vi "Data Channel.vi"(8 "error in (no error)":errorcluster, 11 "Node Ptr":T2 format="%.0x") -> (0 "error out":errorcluster)   [LabVIEW 2019, in "RefMem DMA System Explorer.lvlib"]
uses:
  RefMem DMA System Explorer.lvlib
  <vilib>/NI VeriStand/Custom Device API/Custom Device Item Ref.ctl
  controls/Data Channel Type.ctl
  <vilib>/NI VeriStand/Custom Device API/Custom Device Channel Type.ctl
  Shared/Constants.vi
  <vilib>/NI VeriStand/Custom Device API/Get Item Property (U32).vi
  <vilib>/NI VeriStand/Custom Device API/Get Item Property (U16).vi
  <vilib>/NI VeriStand/Custom Device API/Set Item Property (U32).vi
  <vilib>/NI VeriStand/Custom Device API/Set Item Property (U16).vi
  <vilib>/NI VeriStand/Custom Device API/Custom Device API.lvlib
  Shared/RefMem DMA Shared.lvlib
panel:
  in  "Block Address":u32 format="%.0x"
  in  "Default Value":dbl
  in  "Unit":string
  in  "Warning text":string="WARNING: The address selected by this channel is within the range of addresses reserved by NI VeriStand's built in reflective memory support!"
  out "Warn Icon":bool
  in  "Type":T1
  in  "Relative offset in block":u32
  in  "Header":cluster{"Section Name":string}={"Section Name"="Data Channel"}
  in  "Description":string
  in  "Name":string
  # "In channels (doubles)"
  # "Channels to write has to be in row\nChannels to read can have space in between"
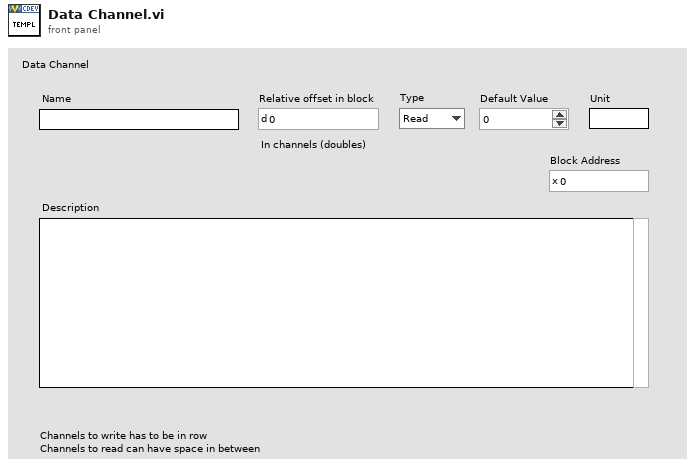
[diagram p1: front panel]
types:
  T1 = typedef "RefMem DMA System Explorer.lvlib/Data Channel Type.ctl" = enum16{"Read", "Write"}
  T2 = typedef "Custom Device API.lvlib/Custom Device Item Ref.ctl" = u64
  T3 = enum8{"Enabled", "Disabled", "Disabled and Grayed Out"}
  T4 = typedef "Custom Device API.lvlib/Custom Device Pointer.ctl" = refnum<k24>
  T5 = typedef "Custom Device API.lvlib/Custom Device Channel.ctl" = cluster{"Type":T6, "Units":string, "Default Value":dbl, "Faultable":bool, "Scalable":bool}
  T6 = typedef "Custom Device API.lvlib/Custom Device Channel Type.ctl" = enum16{"Input", "Output"}
  T7 = typedef "Custom Device API.lvlib/Custom Device Commands.ctl" = enum16{"Default", "Item renamed", "Shutdown", "Dynamic button pressed"}
  T8 = typedef "Custom Device API.lvlib/Custom Device Item Info.ctl" = cluster{"Name":string, "Is Channel":bool, "GUID":string, "Is Waveform":bool}
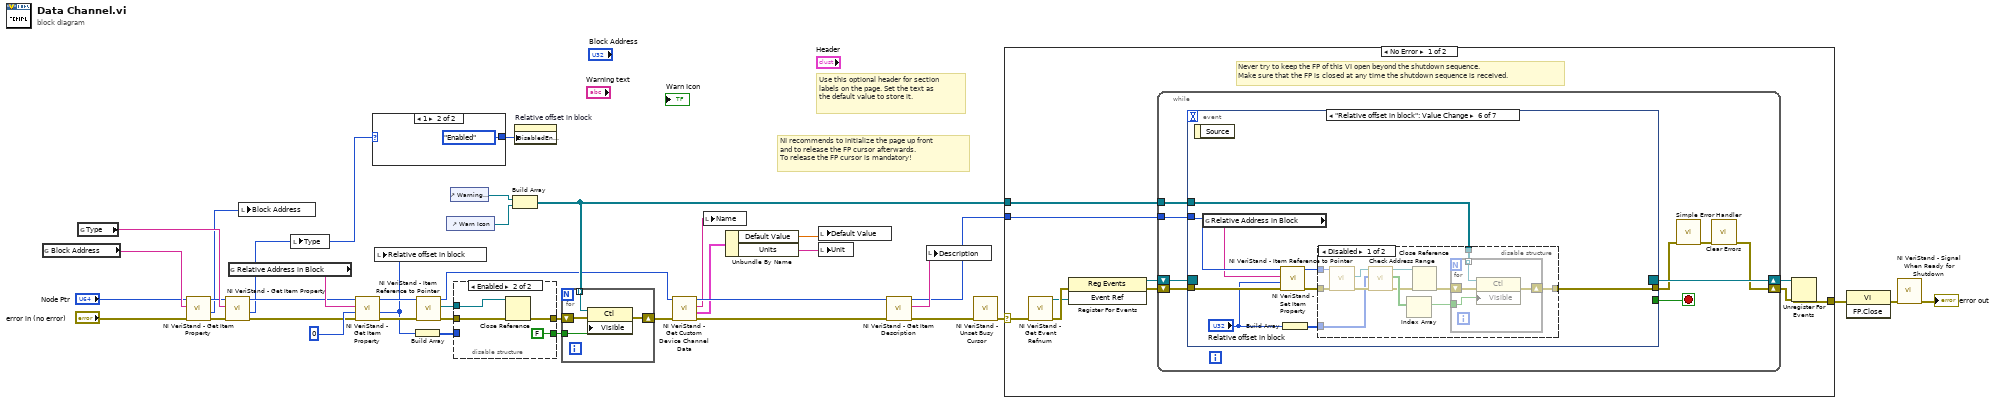
[diagram p0: block diagram]
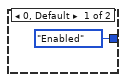
[diagram p2: hidden frame]
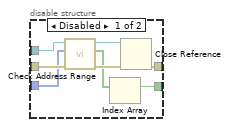
[diagram p3: hidden frame]
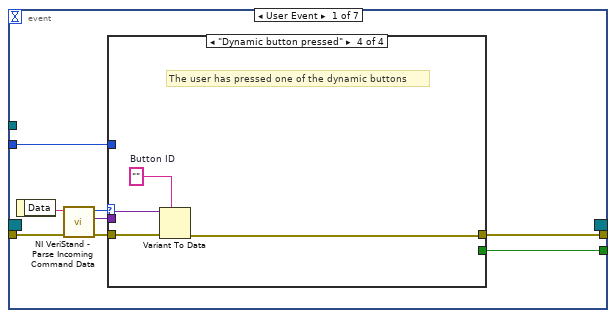
[diagram p4: hidden frame]
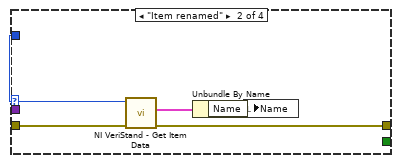
[diagram p6: hidden frame]
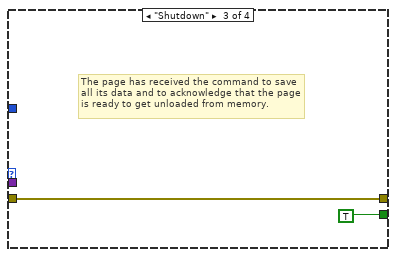
[diagram p7: hidden frame]
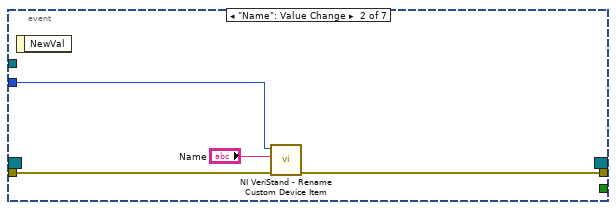
[diagram p8: hidden frame]
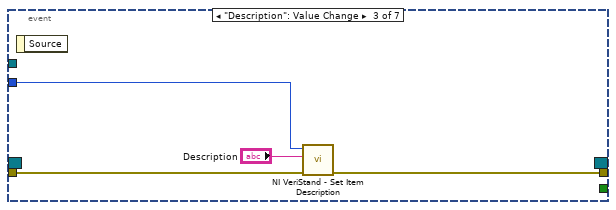
[diagram p9: hidden frame]
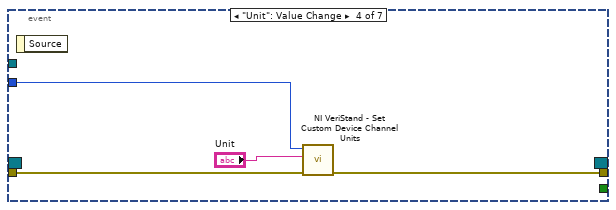
[diagram p10: hidden frame]
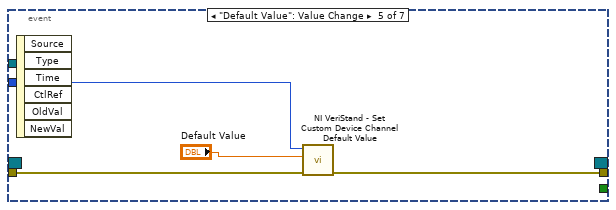
[diagram p11: hidden frame]
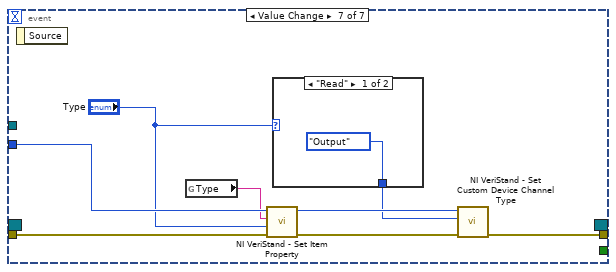
[diagram p13: hidden frame]
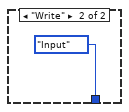
[diagram p14: hidden frame]
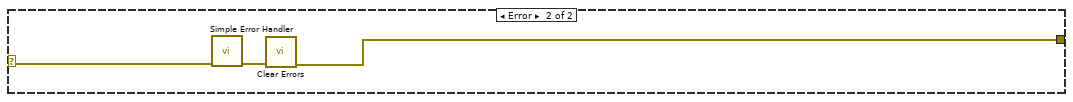
[diagram p15: hidden frame]
diagram:
  # "Use this optional header for section labels on the page. Set the text as the default value to store it."
  # "NI recommends to initialize the page up front\nand to release the FP cursor afterwards.\nTo release the FP cursor is mandatory!"
  n1 = global read "Constants.vi" "Block Address"() -> (w6:string)
  n2 = global read "Constants.vi" "Type"() -> (w21:string)
  n3 = call-poly <vilib>:"NI VeriStand - Get Item Property.vi"("error in (no error)"="error in (no error)", "Property Name"=w6, "Item Ref in"="Node Ptr") -> ("error out"=w7:errorcluster, "Value"=w5:u32, "Item Ref out"=w8:T2)  [unwired: 5 in, 1 out]
  n4 = call-poly <vilib>:"NI VeriStand - Get Item Property.vi"("error in (no error)"=w7, "Property Name"=w21, "Item Ref in"=w8) -> ("error out"=w23:errorcluster, "Value"=w4:u16, "Item Ref out"=w22:T2)  [unwired: 5 in, 1 out]
  n5 = global read "Constants.vi" "Relative Address in Block"() -> (w34:string)
  n6 = local write "Block Address"(w5) -> ()
  n7 = local write "Type"(w4) -> ()
  n8 = call-poly <vilib>:"NI VeriStand - Get Item Property.vi"("error in (no error)"=w23, "Default Value"=u32 0 ("Address"), "Property Name"=w34, "Item Ref in"=w22) -> ("error out"=w32:errorcluster, "Value"=w28:u32, "Item Ref out"=w31:T2)  [unwired: 4 in, 1 out]
  n9 = case shown="1" w4 {
    tunnel: [T3."Enabled" ("Disabled") T3."Enabled" ("Disabled")] -> w3
    frame 0, Default {
    }
    frame 1 {
    }
  }
  n10 = local write "Relative offset in block"(w28) -> ()
  n11 = Build Array(w28) -> (w10:u32[])
  n12 = call <vilib>:"NI VeriStand - Item Reference to Pointer.vi"("error in (no error)"=w32, "Item Ref in"=w31) -> ("error out"=w30:errorcluster, "Node Pointer"=w29:T4, "Item Ref out"=w19:T2)  [unwired: 6 in, 1 out]
  n13 = control-ref of="Warn Icon"() -> (w26:refnum<vi>)
  n14 = control-ref of="Warning text"() -> (w25:refnum<vi>)
  n15 = disable-structure shown="Enabled" {
    disable-tunnel: w30 -> [w49 w52]
    disable-tunnel: w29 -> [w48 w53]
    disable-tunnel: [w45 w51] -> w27
    disable-tunnel: w10 -> [w43 _]
    disable-tunnel: [w42 FALSE ("Inside NIVS Range")] -> w9
    frame Disabled {
      n16 = call "Check Address Range.vi"("error in (no error)"=w49, "Addresses"=w43, "Node Pointer In"=w48) -> ("error out"=w47:errorcluster, "Inside NIVS Range"=w44:bool[], "Node Pointer dup"=w46:T4)  [unwired: 6 in]
      n17 = Index Array(array=w44) -> (element=w42:bool)  [unwired: 1 in]
      n18 = Close Reference(reference=w46, error in (no error)=w47) -> (error out=w45:errorcluster)
    }
    frame Enabled {
      n19 = Close Reference(reference=w53, error in (no error)=w52) -> (error out=w51:errorcluster)
    }
  }
  n20 = Build Array(w25, w26) -> (w24:refnum<vi>[])
  n21 = property on="Relative offset in block" class="DigNum (strict)"("DisabledEnum"=w3) -> ()  [unwired: 2 in, 2 out]
  n22 = for {
    shift-right: [w54] -> w20
    shift-left: w27 -> [w57]
    tunnel: w24 -> [w56] mode=indexing
    tunnel: w9 -> [w55]
    n23 = property on="Property Node" class="Ctl"(reference=w56, error in=w57, "Visible"=w55) -> (error out=w54:errorcluster)  [unwired: 1 out]
  }
  n24 = call <vilib>:"NI VeriStand - Get Custom Device Channel Data.vi"("error in (no error)"=w20, "Channel Ref in"=w19) -> ("error out"=w18:errorcluster, "Channel"=w16:T5, "Channel Name"=w13:string, "Channel Ref out"=w17:T2)  [unwired: 4 in, 2 out]
  n25 = local write "Name"(w13) -> ()
  n26 = Unbundle By Name(w16) -> ("Default Value"=w11:dbl, "Units"=w12:string)
  n27 = local write "Default Value"(w11) -> ()
  n28 = local write "Unit"(w12) -> ()
  n29 = call <vilib>:"NI VeriStand - Get Item Description.vi"("error in (no error)"=w18, "Item Ref in"=w17) -> ("error out"=w15:errorcluster, "Description"=w35:string, "Item Ref out"=w14:T2)  [unwired: 7 out]
  n30 = local write "Description"(w35) -> ()
  n31 = call <vilib>:"NI VeriStand - Unset Busy Cursor.vi"("error in (no error)"=w15) -> ("error out"=w36:errorcluster)  [unwired: 10 out]
  n32 = case shown="No Error" w36 {
    selector: w36 -> [w59 w151]
    tunnel: [w64 w149] -> w39
    tunnel: w14 -> [w60 _]
    tunnel: w24 -> [w58 _]
    frame No Error {
      # "Never try to keep the FP of this VI open beyond the shutdown sequence.\nMake sure that the FP is closed at any time the shutdown sequence is received."
      n33 = call <vilib>:"NI VeriStand - Get Event Refnum.vi"("error in (no error)"=w59) -> ("error out"=w67:errorcluster, "Event Ref"=w63:refnum<user-event>)  [unwired: 9 out]
      n34 = register-events(error in=w67, w63) -> (reference out=w61:refnum<event-registration>, error out=w62:errorcluster)  [unwired: 1 in]
      n35 = while {
        tunnel: w60 -> [w72]
        shift-right: [w69] -> w65
        shift-left: w62 -> [w75]
        shift-right: [w76] -> w66
        shift-left: w61 -> [w74]
        tunnel: w58 -> [w68]
        stop <- w73 stop-if-true
        n36 = event shown="[5] \"Relative offset in block\": Value Change" {
          selector: w74 -> [_ _ _ _ _ _ _]
          dyn-events: [_ _ _ _ _ _ _] -> w76
          timeout: _ -> [_ _ _ _ _ _ _]
          tunnel: w75 -> [w84 w100 w103 w107 w111 w121 w146]
          tunnel: [w80 _ _ _ _ _ _] -> w73
          tunnel: [w79 w99 w102 w106 w110 w114 w141] -> w71
          tunnel: w72 -> [w78 w98 w104 w108 w112 w120 w145]
          tunnel: w68 -> [_ _ _ _ _ w115 _]
          event User Event {
            n37 = event-data() -> ("Data"=w83:string)  [unwired: 1 out]
            n38 = call <vilib>:"NI VeriStand - Parse Incoming Command Data.vi"("error in (no error)"=w84, "Incoming data"=w83) -> ("error out"=w82:errorcluster, "Outgoing data"=w77:variant, "Action"=w81:T7)  [unwired: 7 out]
            n39 = case shown="\"Dynamic button pressed\"" w81 {
              tunnel: w82 -> [w85 w90 w91 w96]
              tunnel: [_ _ TRUE _] -> w80
              tunnel: [w85 w87 w91 w93] -> w79
              tunnel: w78 -> [_ w89 _ _]
              tunnel: w77 -> [_ _ _ w95]
              frame "Default", Default {
              }
              frame "Item renamed" {
                n40 = call <vilib>:"NI VeriStand - Get Item Data.vi"("error in (no error)"=w90, "Item Ref in"=w89) -> ("error out"=w87:errorcluster, "Item Info"=w88:T8)  [unwired: 8 out]
                n41 = Unbundle By Name(w88) -> ("Name"=w86:string)
                n42 = local write "Name"(w86) -> ()
              }
              frame "Shutdown" {
                # "The page has received the command to save all its data and to acknowledge that the page is ready to get unloaded from memory."
              }
              frame "Dynamic button pressed" {
                w94 = ""  # Button ID
                # "The user has pressed one of the dynamic buttons"
                n43 = Variant To Data(error in=w96, type=w94, Variant=w95) -> (error out=w93:errorcluster)  [unwired: 1 out]
              }
            }
          }
          event "Name": Value Change {
            n44 = event-data() -> ()  [unwired: 2 out]
            n45 = call <vilib>:"NI VeriStand - Rename Custom Device Item.vi"("error in (no error)"=w100, "New Name"="Name", "Item Ref in"=w98) -> ("error out"=w99:errorcluster)  [unwired: 1 in, 7 out]
          }
          event "Description": Value Change {
            n46 = event-data() -> ()  [unwired: 2 out]
            n47 = call <vilib>:"NI VeriStand - Set Item Description.vi"("error in (no error)"=w103, "Description"="Description", "Item Ref in"=w104) -> ("error out"=w102:errorcluster)  [unwired: 8 out]
          }
          event "Unit": Value Change {
            n48 = event-data() -> ()  [unwired: 2 out]
            n49 = call <vilib>:"NI VeriStand - Set Custom Device Channel Units.vi"("error in (no error)"=w107, "Units"="Unit", "Channel Ref in"=w108) -> ("error out"=w106:errorcluster)  [unwired: 7 in, 1 out]
          }
          event "Default Value": Value Change {
            n50 = event-data() -> ()  [unwired: 7 out]
            n51 = call <vilib>:"NI VeriStand - Set Custom Device Channel Default Value.vi"("error in (no error)"=w111, "Default Value"="Default Value", "Channel Ref in"=w112) -> ("error out"=w110:errorcluster)  [unwired: 7 in, 1 out]
          }
          event "Relative offset in block": Value Change {
            n52 = event-data() -> ()  [unwired: 2 out]
            n53 = global read "Constants.vi" "Relative Address in Block"() -> (w119:string)
            n54 = call-poly <vilib>:"NI VeriStand - Set Item Property.vi"("error in (no error)"=w121, "Value"="Relative offset in block", "Property Name"=w119, "Item Ref in"=w120) -> ("error out"=w117:errorcluster, "Item Ref out"=w116:T2)  [unwired: 5 in, 1 out]
            n55 = Build Array("Relative offset in block") -> (w113:u32[])
            n56 = disable-structure shown="Disabled" {
              disable-tunnel: w117 -> [w127 w138]
              disable-tunnel: w116 -> [w126 _]
              disable-tunnel: w115 -> [w125 _]
              disable-tunnel: [w124 w138] -> w114
              disable-tunnel: w113 -> [w123 _]
              frame Disabled {
                n57 = call <vilib>:"NI VeriStand - Item Reference to Pointer.vi"("error in (no error)"=w127, "Item Ref in"=w126) -> ("error out"=w128:errorcluster, "Node Pointer"=w129:T4)  [unwired: 6 in, 2 out]
                n58 = call "Check Address Range.vi"("error in (no error)"=w128, "Addresses"=w123, "Node Pointer In"=w129) -> ("error out"=w130:errorcluster, "Inside NIVS Range"=w133:bool[], "Node Pointer dup"=w131:T4)  [unwired: 6 in]
                n59 = Index Array(array=w133) -> (element=w122:bool)  [unwired: 1 in]
                n60 = Close Reference(reference=w131, error in (no error)=w130) -> (error out=w132:errorcluster)
                n61 = for {
                  shift-right: [w134] -> w124
                  shift-left: w132 -> [w137]
                  tunnel: w125 -> [w136] mode=indexing
                  tunnel: w122 -> [w135]
                  n62 = property on="Property Node" class="Ctl"(reference=w136, error in=w137, "Visible"=w135) -> (error out=w134:errorcluster)  [unwired: 1 out]
                }
              }
              frame Enabled {
              }
            }
          }
          event Value Change {
            n63 = event-data() -> ()  [unwired: 2 out]
            n64 = global read "Constants.vi" "Type"() -> (w144:string)
            n65 = call-poly <vilib>:"NI VeriStand - Set Item Property.vi"("error in (no error)"=w146, "Value"="Type", "Property Name"=w144, "Item Ref in"=w145) -> ("error out"=w143:errorcluster, "Item Ref out"=w142:T2)  [unwired: 5 in, 1 out]
            n66 = case shown="\"Read\"" "Type" {
              tunnel: [Custom_Device_Channel_Type."Output" ("Type") Custom_Device_Channel_Type."Input" ("Type")] -> w139
              frame "Read" {
              }
              frame "Write" {
              }
            }
            n67 = call <vilib>:"NI VeriStand - Set Custom Device Channel Type.vi"("error in (no error)"=w143, "Type"=w139, "Channel Ref in"=w142) -> ("error out"=w141:errorcluster)  [unwired: 7 in, 1 out]
          }
        }
        n68 = call <vilib>:"Simple Error Handler.vi"("error in (no error)"=w71) -> ("error out"=w70:errorcluster)  [unwired: 1 in, 7 out]
        n69 = call <vilib>:"Clear Errors.vi"("error in (no error)"=w70) -> ("error out"=w69:errorcluster)  [unwired: 1 in, 5 out]
      }
      n70 = Unregister For Events(event registration refnum=w66, error in=w65) -> (error out=w64:errorcluster)
    }
    frame Error {
      n71 = call <vilib>:"Simple Error Handler.vi"("error in (no error)"=w151) -> ("error out"=w150:errorcluster)  [unwired: 1 in, 7 out]
      n72 = call <vilib>:"Clear Errors.vi"("error in (no error)"=w150) -> ("error out"=w149:errorcluster)  [unwired: 1 in, 5 out]
    }
  }
  n73 = invoke class="VI" method="FP.Close"(error in=w39) -> (error out=w38:errorcluster)  [unwired: 2 in, 2 out]
  n74 = call <vilib>:"NI VeriStand - Signal When Ready for Shutdown.vi"("error in (no error)"=w38) -> ("error out"=→"error out":errorcluster)  [unwired: 10 out]
